vi "GetVITerminalNames.vi"(8 "VI Path":path, 11 "ConNum":i8[](array[numeric])) -> (2 "VI Terminal Names":string[](array[string]))   [LabVIEW 2020]
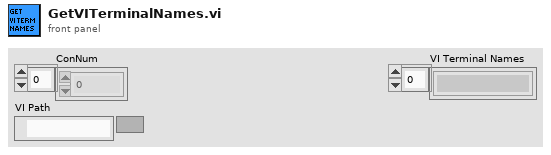
[diagram p1: front panel]
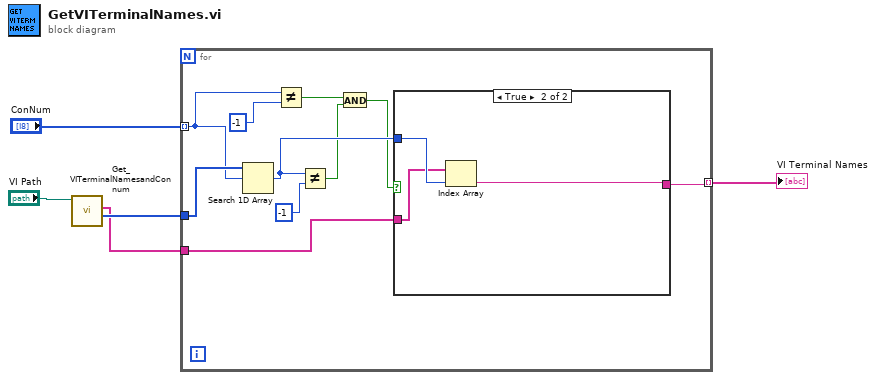
[diagram p0: block diagram]
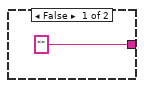
[diagram p2: hidden frame]
diagram:
  n1 = call <vilib>:"Get_VITerminalNamesandConnum.vi"("VI Path"="VI Path") -> ("Connum"=w4:i32[], "VI Terminal Names"=w2:string[])  [unwired: 9 in]
  n2 = for {
    tunnel: w4 -> [w15]
    tunnel: "ConNum" -> [w10] mode=indexing
    tunnel: w2 -> [w13]
    tunnel: [w11] -> w1 mode=indexing
    n3 = Search 1D Array(1D array=w15, element=w10) -> (index of element=w12:i32)  [unwired: 1 in]
    n4 = Not Equal?(x=w10, y=-1) -> (x != y?=w9:bool)
    n5 = Not Equal?(x=w12, y=-1) -> (x != y?=w8:bool)
    n6 = And(x=w9, y=w8) -> (x .and. y?=w7:bool)
    n7 = case shown="True" w7 {
      tunnel: w13 -> [_ w18]
      tunnel: w12 -> [_ w19]
      tunnel: ["" ("Name") w17] -> w11
      frame False {
      }
      frame True {
        n8 = Index Array(array=w18, index=w19) -> (element=w17:string)
      }
    }
  }
  "VI Terminal Names" <- w1
